vi "File-IO-test.vi"(0 "Chan":string="Vibration", 1 "Operation":T1, 5 "Vibration Channel Name Input":string[](array[string]), 7 "文件路径":path, 9 "Test Info":cluster{"Test Name":string, "Tester":string} caption="Test Information Input", 11 "Vibration Waveform":waveform(dbl)[](array[waveform]), 12 "error in":errorcluster caption="Error In") -> (4 "通道名":string[](array[string]), 8 "Vibration Waveform out":waveform(dbl)[](array[waveform]), 10 "Test Info 2":cluster{"Test Name":string, "Tester":string} caption="Test Information Output", 15 "error out":errorcluster caption="Error out")   [LabVIEW 2011]
panel:
  in  "GroupName":string="TEST DATA"
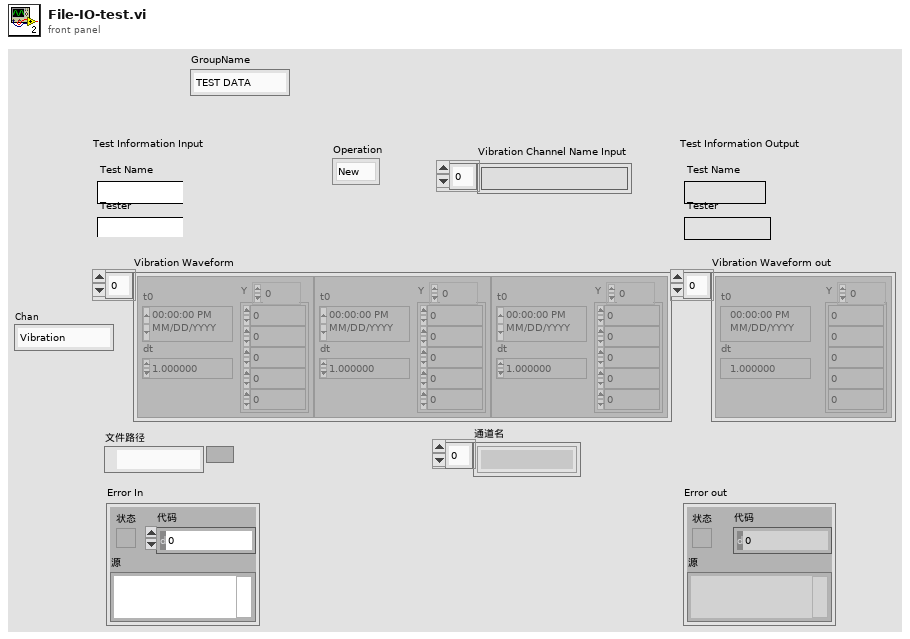
[diagram p1: front panel]
types:
  T1 = typedef "Enum File IO - FGV(V)_Ctrls-某型振动实验台测试系统.ctl" = enum16{"New", "Open", "Write Info", "Write Data", "Read Info", "Read Chan Names", "Read Data", "Close", "None"}
  T2 = enum16{"open", "open or create", "create or replace", "create", "open (read-only)"}
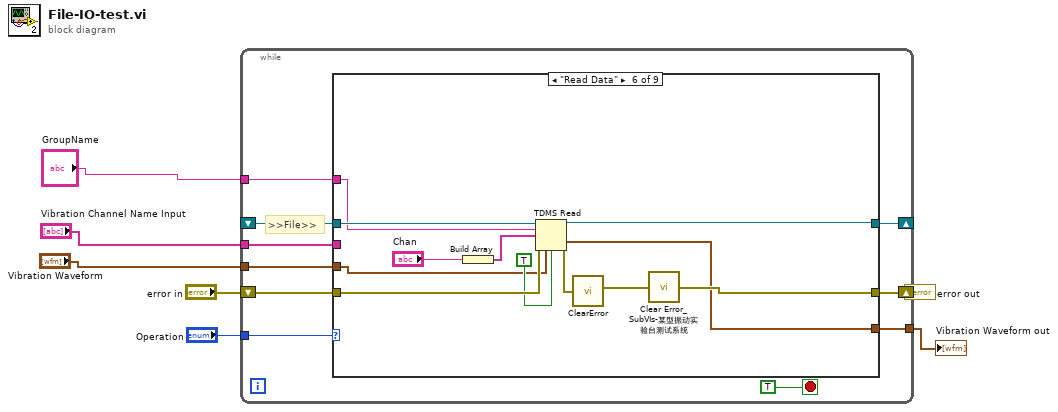
[diagram p0: block diagram]
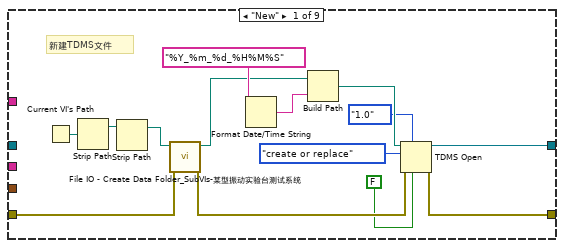
[diagram p2: hidden frame]
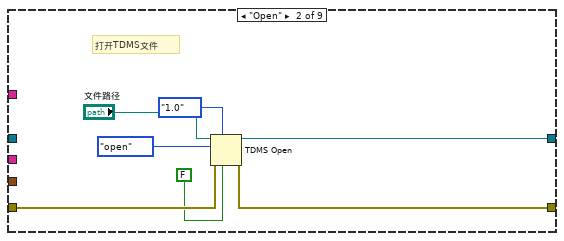
[diagram p3: hidden frame]
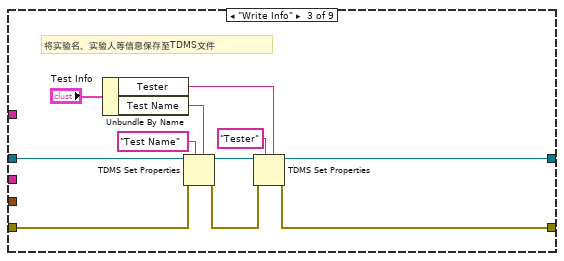
[diagram p4: hidden frame]
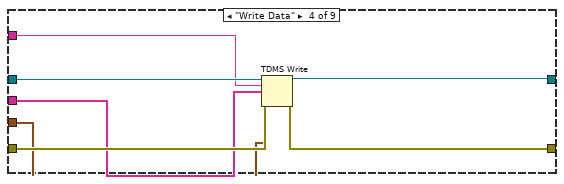
[diagram p5: hidden frame]
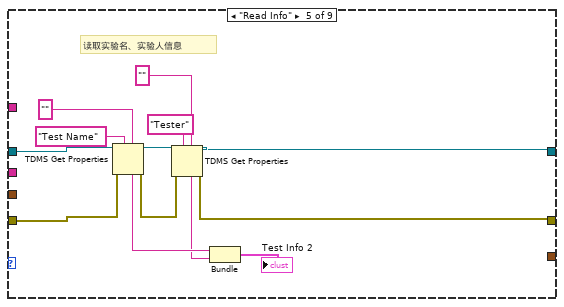
[diagram p6: hidden frame]
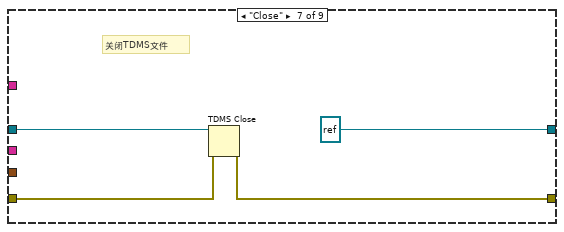
[diagram p7: hidden frame]
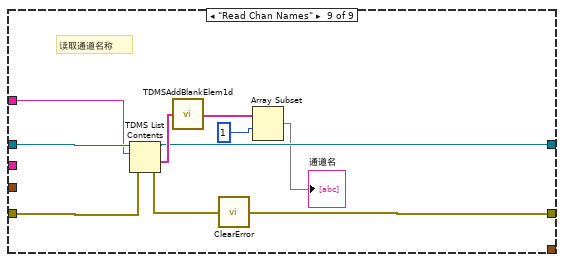
[diagram p9: hidden frame]
diagram:
  n1 = while {
    tunnel: "Operation" -> [w16]
    shift-right: [w14] -> w5
    shift-left: "error in" -> [w13]
    shift-right: [w15] -> _
    shift-left: _ -> [w12]
    tunnel: "Vibration Channel Name Input" -> [w10]
    tunnel: "Vibration Waveform" -> [w9]
    tunnel: "GroupName" -> [w8]
    tunnel: [w11] -> w4
    stop <- TRUE stop-if-true
    # ">>File>>"
    n2 = case shown="\"Read Data\"" w16 {
      tunnel: [w31 w36 w40 w54 w58 w79 refnum<k34> refnum ("tdms file out") w87 w91] -> w15
      tunnel: [w28 w37 w39 w53 w57 w78 w82 w86 w95] -> w14
      tunnel: w13 -> [w24 w38 w49 w55 w69 w80 w85 w86 w96]
      tunnel: w12 -> [_ _ w48 w56 w61 w81 w84 w87 w97]
      tunnel: [_ _ _ _ _ w74 _ _ _] -> w11
      tunnel: w10 -> [_ _ _ w52 _ _ _ _ _]
      tunnel: w9 -> [_ _ _ w51 _ w72 _ _ _]
      tunnel: w8 -> [_ _ _ w50 _ w73 _ _ w93]
      frame "New" {
        # "新建TDMS文件"
        n3 = Current VI's Path() -> (path=w26:path)
        n4 = Strip Path(path=w26) -> (stripped path=w25:path)  [unwired: 1 out]
        n5 = Strip Path(path=w25) -> (stripped path=w23:path)  [unwired: 1 out]
        n6 = call "File IO - Create Data Folder_SubVIs-某型振动实验台测试系统.vi"("error in"=w24, "path input"=w23) -> ("error out"=w22:errorcluster, "path output"=w21:path)  [unwired: 8 out]
        n7 = Format Date/Time String(time format string (%c)="%Y_%m_%d_%H%M%S" ("时间格式字符串(%c)")) -> (date/time string=w20:string)  [unwired: 2 out]
        n8 = Build Path(base path=w21, name or relative path=w20) -> (appended path=w29:path)
        n9 = TDMS Open(6:FALSE ("禁用缓存(T)"), 7:enum16{"1.0", "2.0"}."1.0" ("文件格式版本(2.0)"), 8:w22, 10:T2."create or replace" ("操作(0:open)"), 11:w29) -> (0:w28:errorcluster, 3:w31:refnum<k34>)  [unwired: 1 in]
      }
      frame "Open" {
        # "打开TDMS文件"
        n10 = TDMS Open(6:FALSE ("禁用缓存(T)"), 7:enum16{"1.0", "2.0"}."1.0" ("文件格式版本(2.0)"), 8:w38, 10:T2."open" ("操作(0:open)"), 11:"文件路径") -> (0:w37:errorcluster, 3:w36:refnum<k34>)  [unwired: 1 in]
      }
      frame "Write Info" {
        # "将实验名、实验人等信息保存至TDMS文件"
        n11 = Unbundle By Name("Test Info") -> ("Tester"=w41:string, "Test Name"=w42:string)
        n12 = TDMS Set Properties(5:w42, 7:"Test Name", 8:w49, 11:w48) -> (0:w46:errorcluster, 3:w45:refnum<k34>)  [unwired: 4 out]
        n13 = TDMS Set Properties(5:w41, 7:"Tester", 8:w46, 11:w45) -> (0:w39:errorcluster, 3:w40:refnum<k34>)  [unwired: 4 out]
      }
      frame "Write Data" {
        n14 = TDMS Write(0:w56, 5:w50, 7:w52, 9:w51, 11:w55) -> (4:w54:refnum<k34>, 15:w53:errorcluster)  [unwired: 1 in, 2 out]
      }
      frame "Read Info" {
        # "读取实验名、实验人信息"
        n15 = TDMS Get Properties(5:"", 7:"Test Name", 8:w69, 11:w61) -> (0:w68:errorcluster, 3:w60:refnum<k34>, 4:w63:string)  [unwired: 5 out]
        n16 = TDMS Get Properties(5:"", 7:"Tester", 8:w68, 11:w60) -> (0:w57:errorcluster, 3:w58:refnum<k34>, 4:w59:string)  [unwired: 5 out]
        n17 = Bundle(w63, w59) -> (→"Test Info 2":cluster{string, string})  [unwired: 1 out]
      }
      frame "Read Data" {
        n18 = Build Array("Chan") -> (w70:string[])
        n19 = TDMS Read(0:w81, 5:w73, 7:w70, 11:w80, 12:w72, 13:TRUE ("return channels in file order? (F)")) -> (4:w79:refnum<k34>, 10:w74:waveform(dbl)[], 15:w76:errorcluster)  [unwired: 2 in, 3 out]
        n20 = call <vilib>:"ClearError.vi"("error in (no error)"=w76) -> ("error out"=w77:errorcluster)
        n21 = call "Clear Error_SubVIs-某型振动实验台测试系统.vi"("error in (no error)"=w77) -> ("error out"=w78:errorcluster)
      }
      frame "Close" {
        # "关闭TDMS文件"
        n22 = TDMS Close(8:w85, 11:w84) -> (0:w82:errorcluster)  [unwired: 1 out]
      }
      frame "None", Default {
      }
      frame "Read Chan Names" {
        # "读取通道名称"
        n23 = TDMS List Contents(4:w96, 6:w93, 7:w97) -> (0:w94:errorcluster, 1:w92:string[], 3:w91:refnum<k34>)  [unwired: 1 out]
        n24 = call <vilib>:"TDMSAddBlankElem1d.vi"("input string array"=w92) -> ("output string array with blank element at the beginning"=w90:string[])
        n25 = call <vilib>:"ClearError.vi"("error in (no error)"=w94) -> ("error out"=w95:errorcluster)
        n26 = Array Subset(array=w90, index=1 ("索引")) -> (→"通道名":string[])  [unwired: 1 in]
      }
    }
  }
  "error out" <- w5
  "Vibration Waveform out" <- w4
